vi "Add-log-message-simple.vi"(8 "error in (no error)":errorcluster, 10 "Message":string, 11 "UI in":T1) -> (0 "error out":errorcluster, 3 "UI out":T1)   [LabVIEW 2013, in "PowderDeposition.lvlib" / "PD-Main.lvclass"]
uses:
  PD-Main.lvclass
  Object-reference.ctl
  PD-Main.lvclass/PD-Main.ctl
  Read Activity log.vi
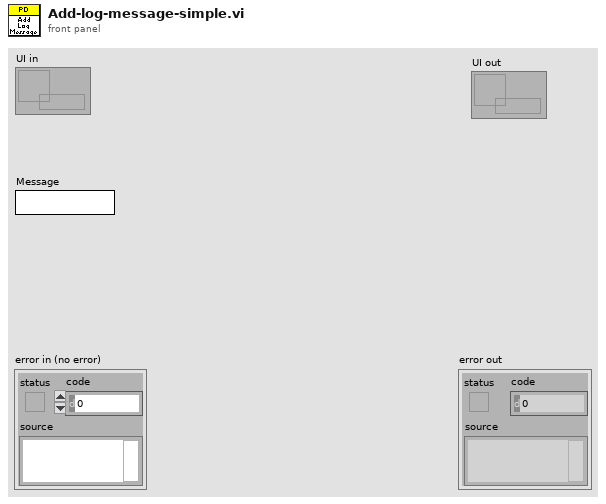
[diagram p1: front panel]
types:
  T1 = typedef "PowderDeposition.lvlib/PD-Main.lvclass/Object-reference.ctl" = refnum<data-value>
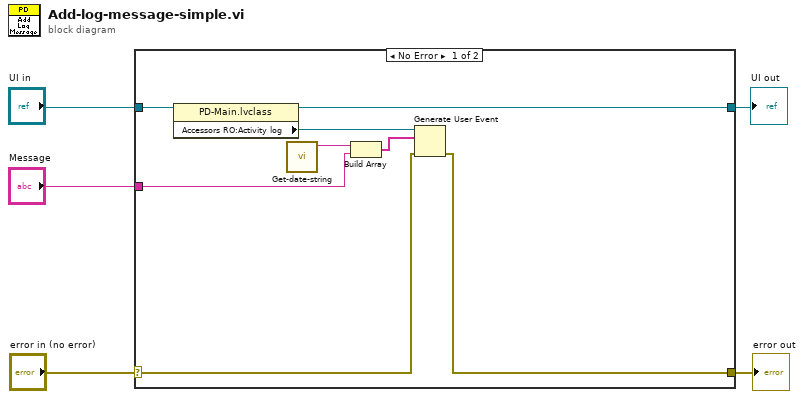
[diagram p0: block diagram]
diagram:
  n1 = case shown="No Error" "error in (no error)" {
    selector: "error in (no error)" -> [w9 w15]
    tunnel: [w8 w15] -> w4
    tunnel: [w7 w14] -> w1
    tunnel: "UI in" -> [w11 w14]
    tunnel: "Message" -> [w12 _]
    frame No Error {
      n2 = property class="PD-Main.lvclass"(reference=w11) -> (reference out=w7:T1, "Accessors RO:Activity log"=w6:refnum<user-event>)  [unwired: 1 in, 1 out]
      n3 = call "Get-date-string.vi"() -> ("Date string"=w13:string)  [unwired: 11 in]
      n4 = Build Array(w13, w12) -> (w10:string[])
      n5 = Generate User Event(user event=w6, event data cluster=w10, error in=w9) -> (error out=w8:errorcluster)  [unwired: 1 in, 1 out]
    }
    frame Error {
    }
  }
  "error out" <- w4
  "UI out" <- w1
